vi "ProdaNG.WabcoPartProcesses.Get.vi"(8 "error in (no error)":errorcluster, 10 "WabcoPartId":i32, 11 "dbHandleIn":i32) -> (0 "error out":errorcluster, 2 "Proc":T1[](array[typedef]), 3 "dbHandle":i32)   [LabVIEW 2016]
doc: "This function returns a product structure for a product, which is identified by a part and a serial number.\nImportant information: The field 'individual' was taken over from the field 'allgemein' of the legacy data directly. Because of this most products have the value 0 further on and only a few the value 1. \nParameter:\nhandle is an Integer, which is returned by the function Login() at the creation of a new connection.\nwabcoPartId is the Id of the part.\nserialNumber is the serial number of the product for the part above.\nproduct is a pointer on a product structure, which is filled if the returncode is 0. The structure must be defined in the calling program.\n\nReturncodes:\n0 No error\n< 0 ORACLE Error code\n6 (ERROR_INVALID_HANDLE) in case of an invalid handle\n1403 Record does not exist"
uses:
  Controls/ProdaNG.Process.ctl
  Controls/ProdaNG.ProcessSize.ctl
  <vilib>/Utility/importsl/GetValueByPointer/datatype.ctl
  <vilib>/Utility/importsl/GetValueByPointer/GetValueByPointer.xnode
  prodllNG.dll
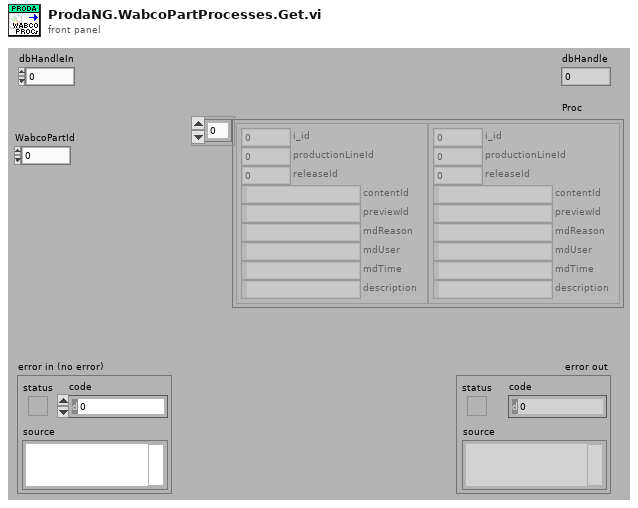
[diagram p1: front panel]
types:
  T1 = typedef "ProdaNG.Process.ctl" = cluster{"i_id":i32, "productionLineId":i32, "releaseId":i32, "contentId":string, "previewId":string, "mdReason":string, "mdUser":string, "mdTime":string, "description":string}
  T2 = typedef "ProdaNG.ProcessSize.ctl" = cluster{"i_id":i32, "productionLineId":i32, "releaseId":i32, "contentId":i32, "previewId":i32, "mdReason":i32, "mdUser":i32, "mdTime":i32, "description":i32}
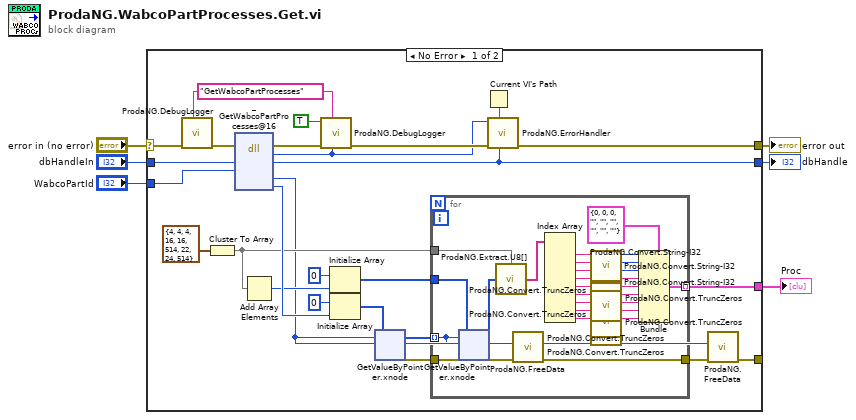
[diagram p0: block diagram]
diagram:
  n1 = case shown="No Error" "error in (no error)" {
    selector: "error in (no error)" -> [w27 w92]
    tunnel: [w32 w92] -> w5
    tunnel: "dbHandleIn" -> [w29 w91]
    tunnel: [w30 w91] -> w3
    tunnel: [w12 _] -> w2
    tunnel: [w9 _] -> _
    tunnel: "WabcoPartId" -> [w7 _]
    frame No Error {
      w23 = "GetWabcoPartProcesses" ("cmd")
      n2 = call "ProdaNG.DebugLogger.vi"("cmd"=w23, "error in (no error)"=w27) -> ("error out"=w26:errorcluster)  [unwired: 9 in]
      n3 = Cluster To Array(cluster=T2 {"i_id"=4, "productionLineId"=4, "releaseId"=4, "contentId"=16, "previewId"=16, "mdReason"=514, "mdUser"=22, "mdTime"=24, "description"=514} ("ProcSize")) -> (array=w13:i32[])
      n4 = dll-call lib="D:/svn/LineTraceSystem/SOFTWARE/sources/Database/ProdaNG/prodllNG.dll" fn="_GetWabcoPartProcesses@16" ("ProDLL wrapper.dll:ProDLL_wrapper_GetWabcoParts_GetData")(error in=w26, "dbHandle"=w29, "WabcoPartId"=w7) -> (error out=w25:errorcluster, "return type"=w22:i32, "dbHandle"=w30:i32, "processesPtr"=w10:u32, "countPtr"=w17:i32)  [unwired: 5 in, 1 out]
      n5 = Add Array Elements(numeric array=w13) -> (sum=w14:i32)
      n6 = call "ProdaNG.DebugLogger.vi"("return type"=w22, "cmd"=w23, "error in (no error)"=w25, "done? (F)"=TRUE) -> ("error out"=w24:errorcluster)  [unwired: 7 in]
      n7 = Initialize Array(u8 0 ("element"), w14) -> (w15:u8[])
      n8 = Initialize Array(u32 0 ("element"), w17) -> (w21:u32[])
      n9 = xnode "GetValueByPointer.xnode"("Pointer"=w10, "InputType"=w21) -> ("Output"=w18:u32[], "ErrorOut"=w19:errorcluster)  [unwired: 2 in]
      n10 = for {
        tunnel: w19 -> [w60]
        tunnel: w18 -> [w42] mode=indexing
        tunnel: w15 -> [w59]
        tunnel: w13 -> [w48]
        tunnel: [w47] -> w12 mode=indexing
        tunnel: [w40] -> w11
        n11 = xnode "GetValueByPointer.xnode"("Pointer"=w42, "InputType"=w59, "ErrorIn"=w60) -> ("Output"=w50:u8[], "ErrorOut"=w41:errorcluster)  [unwired: 1 in]
        n12 = call "ProdaNG.Extract.U8[].vi"("unsigned byte array"=w50, "Sizes"=w48) -> ("Elements"=w49:string[])
        n13 = call "ProdaNG.FreeData.vi"("error in (no error)"=w41, "Pointers"=w42) -> ("error out"=w40:errorcluster)  [unwired: 9 in]
        n14 = Index Array(array=w49) -> (element #1=w52:string, element #2=w51:string, element #3=w34:string, element #4=w38:string, element #5=w56:string, element #6=w58:string, element #7=w46:string, element #8=w45:string, element #9=w35:string)  [unwired: 9 in]
        n15 = call "ProdaNG.Convert.String-I32.vi"("unsigned byte string"=w52) -> ("32bit integer"=w54:i32)  [unwired: 10 in]
        n16 = call "ProdaNG.Convert.String-I32.vi"("unsigned byte string"=w51) -> ("32bit integer"=w53:i32)  [unwired: 10 in]
        n17 = call "ProdaNG.Convert.String-I32.vi"("unsigned byte string"=w34) -> ("32bit integer"=w33:i32)  [unwired: 10 in]
        n18 = call "ProdaNG.Convert.TruncZeros.vi"("string with \\0s"=w38) -> ("LV string"=w37:string)  [unwired: 10 in]
        n19 = call "ProdaNG.Convert.TruncZeros.vi"("string with \\0s"=w56) -> ("LV string"=w55:string)  [unwired: 10 in]
        n20 = call "ProdaNG.Convert.TruncZeros.vi"("string with \\0s"=w58) -> ("LV string"=w57:string)  [unwired: 10 in]
        n21 = call "ProdaNG.Convert.TruncZeros.vi"("string with \\0s"=w46) -> ("LV string"=w44:string)  [unwired: 10 in]
        n22 = call "ProdaNG.Convert.TruncZeros.vi"("string with \\0s"=w45) -> ("LV string"=w43:string)  [unwired: 10 in]
        n23 = call "ProdaNG.Convert.TruncZeros.vi"("string with \\0s"=w35) -> ("LV string"=w36:string)  [unwired: 10 in]
        n24 = Bundle(cluster=T1 {"i_id"=0, "productionLineId"=0, "releaseId"=0, "contentId"="", "previewId"="", "mdReason"="", "mdUser"="", "mdTime"="", "description"=""} ("ProcessStep"), "i_id"=w54, "productionLineId"=w53, "releaseId"=w33, "contentId"=w37, "previewId"=w55, "mdReason"=w57, "mdUser"=w44, "mdTime"=w43, "description"=w36) -> (w47:T1)
      }
      n25 = Current VI's Path() -> (path=w31:path)
      n26 = call "ProdaNG.ErrorHandler.vi"("dbHandleIn"=w30, "Path"=w31, "error in"=w24, "output_parameter"=w22) -> ("error out"=w32:errorcluster)  [unwired: 7 in]
      n27 = call "ProdaNG.FreeData.vi"("error in (no error)"=w11, "Pointers"=w10) -> ("error out"=w9:errorcluster)  [unwired: 9 in]
    }
    frame Error {
    }
  }
  "error out" <- w5
  "dbHandle" <- w3
  "Proc" <- w2
